vi "Populate Serial Channels.vi"(8 "error in (no error)":errorcluster, 10 "Strings []":string[](array[string]), 11 "SERIAL INPUT (SI) Ref in":refnum<vi>) -> (0 "error out":errorcluster, 3 "SERIAL INPUT (SI) Ref out":refnum<vi>)   [LabVIEW 2025, in "I2C Bus Monitor UI.lvlib"]
uses:
  I2C Bus Monitor UI.lvlib
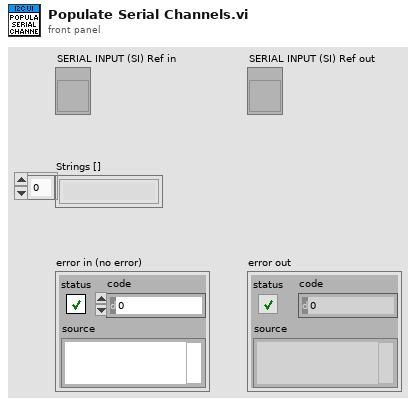
[diagram p1: front panel]
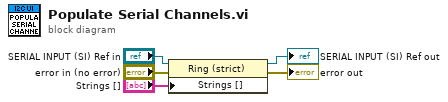
[diagram p0: block diagram]
diagram:
  n1 = property on="Property Node" class="Ring (strict)"(reference="SERIAL INPUT (SI) Ref in", error in="error in (no error)", "Strings []"="Strings []") -> (reference out=→"SERIAL INPUT (SI) Ref out":refnum<vi>, error out=→"error out":errorcluster)
